vi "Queue Nested.vi"(8 "Alias":string, 9 "Priority?":bool, 10 "Msg Strategy":refnum<class "Msg.lvclass">, 11 "Base Queue jettl in":refnum<class "Base Queue jettl.lvclass">) -> (3 "Base Queue jettl out":refnum<class "Base Queue jettl.lvclass">)   [LabVIEW 2021, in "jettl.lvlib" / "Base Queue jettl.lvlib" / "Base Queue jettl.lvclass"]
uses:
  Base Queue jettl.lvclass
  Msg Strategy/Msg/Msg.lvclass
  Base Queue jettl.lvclass/Base Queue jettl.ctl
  jettl.lvlib
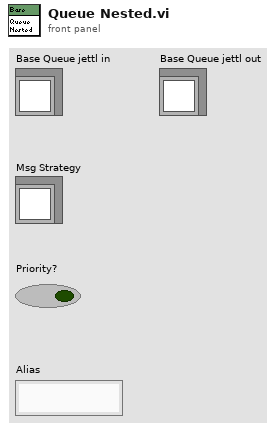
[diagram p1: front panel]
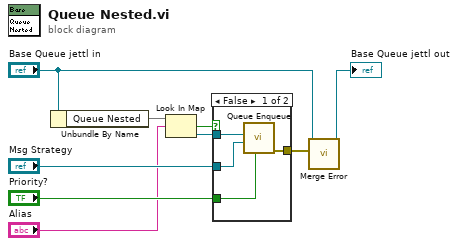
[diagram p0: block diagram]
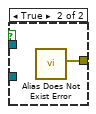
[diagram p2: hidden frame]
diagram:
  n1 = Unbundle By Name("Base Queue jettl in") -> ("Queue Nested"=w5:map{string, refnum<data-value>})
  n2 = Look In Map(map=w5, key="Alias") -> (key not found?=w4:bool, value=w7:refnum<data-value>)  [unwired: 1 in]
  n3 = case shown="False" w4 {
    tunnel: [w13 w14] -> w1
    tunnel: "Priority?" -> [w12 _]
    tunnel: "Msg Strategy" -> [w11 _]
    tunnel: w7 -> [w10 _]
    frame False {
      n4 = call "Queue Enqueue.vi"("Priority?"=w12, "Msg Strategy"=w11, "Queue"=w10) -> ("error out"=w13:errorcluster)  [unwired: 8 in]
    }
    frame True {
      n5 = call "Alias Does Not Exist Error.vi"() -> ("Error"=w14:errorcluster)  [unwired: 11 in]
    }
  }
  n6 = call-dynamic "Merge Error.vi"("Error"=w1, "Base Queue jettl in"="Base Queue jettl in") -> ("Base Queue jettl out"=→"Base Queue jettl out":refnum<class "Base Queue jettl.lvclass">)  [unwired: 9 in]
